vi "show compatible FPGA resources.vi"(9 "Array":variant[](array[variant]), 10 "resource":i32, 11 "TreeControl in":refnum<vi>) -> ()   [LabVIEW 2016, in "FPGA Addon System Explorer.lvlib"]
uses:
  FPGA Addon System Explorer.lvlib
  <vilib>/NI Veristand/Custom Device API/Custom Device Item Ref.ctl
  FPGA-Resource-Manager-APIs/Source/fpga resource.ctl
  FPGA-Resource-Manager-APIs/Source/Channel Type.ctl
  FPGA-Resource-Manager-APIs/Source/System Definition/FPGA RM System Definition API.lvlib
  <vilib>/NI VeriStand/Custom Device API/Custom Device API.lvlib
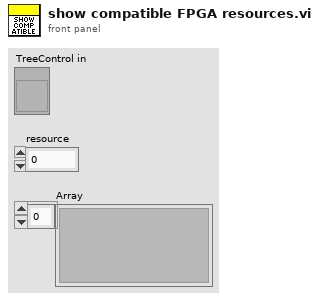
[diagram p1: front panel]
types:
  T1 = cluster{"Left Cell String":string, "Child Text":string[], "Child Tag":string, "Item Indent":i32, "Child Only?":bool, "Glyph Index":i32}
  T2 = typedef "Custom Device API.lvlib/Custom Device Item Ref.ctl" = u64
  T3 = typedef "FPGA RM System Definition API.lvlib/fpga resource.ctl" = cluster{"name":string, "datatype":string, "channel type":T4, "value":variant, "notes":string}
  T4 = typedef "FPGA RM System Definition API.lvlib/Channel Type.ctl" = enum16{"Write Channel", "Read Channel", "Write Waveform", "Read Waveform"}
  T5 = cluster{"Left Cell String":string, "Child Text":string[], "Child Tag":string, "Item Indent":i32, "Child Only?":bool, "Glyph Index":i32}[]
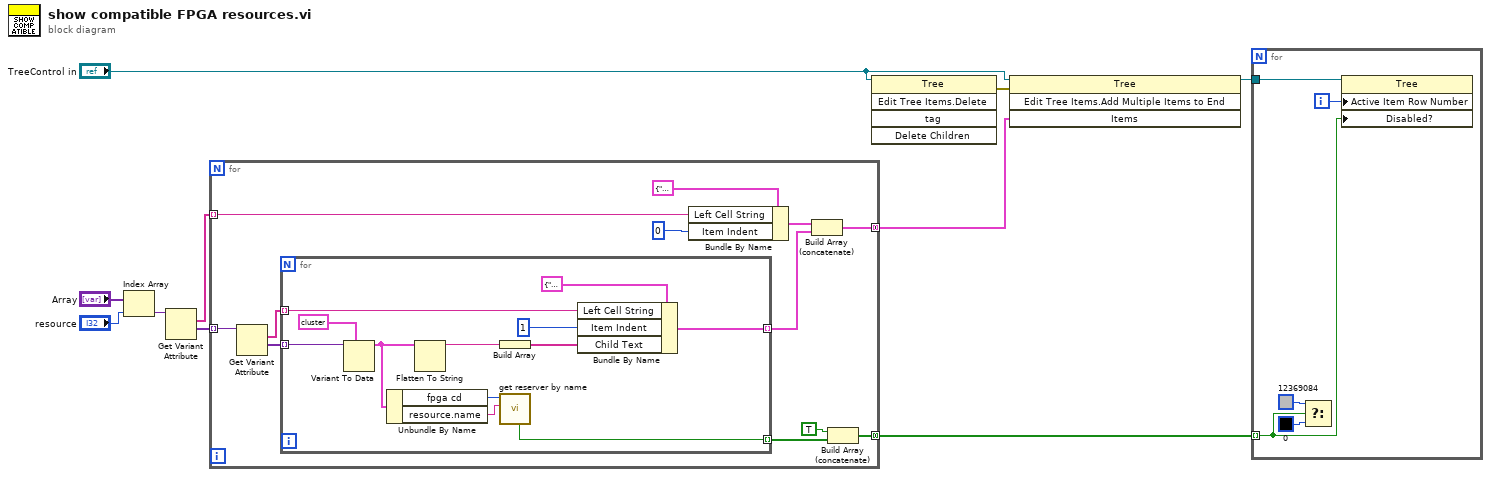
[diagram p0: block diagram]
diagram:
  n1 = Index Array(array="Array", index="resource") -> (element=w6:variant)
  n2 = Get Variant Attribute(Variant=w6) -> (names=w7:string[], values=w8:variant[])  [unwired: 3 in, 2 out]
  n3 = for {
    tunnel: w7 -> [w21] mode=indexing
    tunnel: w8 -> [w19] mode=indexing
    tunnel: [w15] -> w9 mode=concatenating
    tunnel: [w11] -> w2 mode=concatenating
    n4 = Get Variant Attribute(Variant=w19) -> (names=w18:string[], values=w12:variant[])  [unwired: 3 in, 2 out]
    n5 = for {
      tunnel: w18 -> [w32] mode=indexing
      tunnel: [w31] -> w17 mode=indexing
      tunnel: [w26] -> w13 mode=indexing
      tunnel: w12 -> [w30] mode=indexing
      n6 = Variant To Data(type=cluster{"fpga cd":T2, "resource":T3} {"fpga cd"=0, "resource"={"name"="", "datatype"="", "channel type"=enum."Write Channel", "value"=variant, "notes"=""}} ("fpga resources"), Variant=w30) -> (data=w25:cluster{"fpga cd":T2, "resource":T3})  [unwired: 1 in, 1 out]
      n7 = Unbundle By Name(w25) -> ("fpga cd"=w27:T2, "resource.name"=w28:string)
      n8 = Flatten To String(anything=w25) -> (data string=w24:string)  [unwired: 3 in, 2 out]
      n9 = Build Array(w24) -> (w23:string[])
      n10 = call "get reserver by name.vi"("name"=w28, "Item Ref in"=w27) -> ("Found"=w26:bool)  [unwired: 6 in, 3 out]
      n11 = Bundle By Name(cluster=T1 {"Left Cell String"="", "Child Text"=[], "Child Tag"="", "Item Indent"=0, "Child Only?"=FALSE, "Glyph Index"=0} ("Items"), "Left Cell String"=w32, "Item Indent"=1, "Child Text"=w23) -> (w31:T1)
    }
    n12 = Bundle By Name(cluster=T1 {"Left Cell String"="", "Child Text"=[], "Child Tag"="", "Item Indent"=0, "Child Only?"=FALSE, "Glyph Index"=0} ("Items"), "Left Cell String"=w21, "Item Indent"=0) -> (w16:T1)
    n13 = Build Array (concatenate)(w16, w17) -> (w15:T5)
    n14 = Build Array (concatenate)(TRUE, w13) -> (w11:bool[])
  }
  n15 = invoke on="Invoke Node" class="Tree" method="Edit Tree Items.Delete"(reference="TreeControl in") -> (error out=w10:errorcluster)  [unwired: 4 in, 4 out]
  n16 = invoke on="Invoke Node" class="Tree" method="Edit Tree Items.Add Multiple Items to End"(reference="TreeControl in", error in=w10, "Items"=w9) -> (reference out=w1:refnum<vi>)  [unwired: 1 in, 3 out]
  n17 = for {
    tunnel: w2 -> [w35] mode=indexing
    tunnel: w1 -> [w37]
    i -> [w36]
    n18 = Select(t=u32 12369084 ("Active Cell:Cell Font:Color"), s=w35, f=u32 0 ("Active Cell:Cell Font:Color")) -> ()  [unwired: 1 out]
    n19 = property class="Tree"(reference=w37, "Active Item Row Number"=w36, "Disabled?"=w35) -> ()  [unwired: 1 in, 2 out]
  }
